vi "GDSAPI_CreateClass.vi"(7 "KeepLvClassRefOpen(False)":bool, 8 "error in (no error)":errorcluster, 9 "ClassIcon(Random colors are used if not wired)":T1, 10 "CreateClassType":T3={"ClassProvider"=enum."GOOP-3(By reference)", "NewClassFolder"=path "", "ParentLvClassFilePath"=path "", "ClassName"="", "ClassDescription"="", "ClassTemplate"=enum."Standard"}, 11 "ProjectItemToCraeteClassUnder":refnum<vi>) -> (0 "error out":errorcluster, 2 "LVClassLibraryRefnum":refnum<vi>, 3 "LvClassFileOut":path)   [LabVIEW 2016]
doc: "NOT Yet implemented"
uses:
  <resource>/Framework/Providers/Open_GDS/API/GDSAPI_CreateClassType.ctl
  <resource>/Framework/Providers/Open_GDS/API/GDSAPI_SubVIs/GDSAPI_ClassProviderType.ctl
  <resource>/Framework/Providers/Open_GDS/API/GDSAPI_SubVIs/GDSAPI_ClassTemplateType.ctl
  <resource>/Framework/Providers/Open_GDS/API/GDSAPI_SubVIs/GDSAPI_ClassIcon.ctl
  <resource>/Framework/Providers/Open_GDS/API/GDSAPI_SubVIs/GDSAPI_ClassIconType.ctl
  <resource>/Framework/Providers/Open_GDS/ClassProviders/Provider_BaseClassInterface/CreateClassData.ctl
  <resource>/Framework/Providers/Open_GDS/ClassProviders/Common/LvIcon_class/GDSLvIcon_ClassColorTypes.ctl
  <resource>/Framework/Providers/Open_GDS/ClassProviders/Common/ScriptingFunctions/Scripting_ConnectorPanePatternType.ctl
  <resource>/Framework/Providers/Open_GDS/ClassProviders/Provider_LvNativeClass/ClassWriterNative_class/ClassWriterNative.lvclass
  <resource>/Framework/Providers/Open_GDS/ClassProviders/Provider_EndevoGOOP300/ClassWriterGOOP300_class/ClassWriterGOOP300.lvclass
  C:/Program Files (x86)/National Instruments/LabVIEW 2016/resource/Framework/Providers/Open_GDS/ClassProviders/Provider_LvNativeClass/ClassWriterNative_class/ClassWriterNative.lvclass
  <resource>/Framework/Providers/Open_GDS/ClassProviders/Provider_EndevoGOOP400/ClassWriterGOOP400_class/ClassWriterGOOP400.lvclass
  <resource>/Framework/Providers/Open_GDS/ClassProviders/Provider_BaseClassInterface/ClassWriter_class/ClassWriter.lvclass
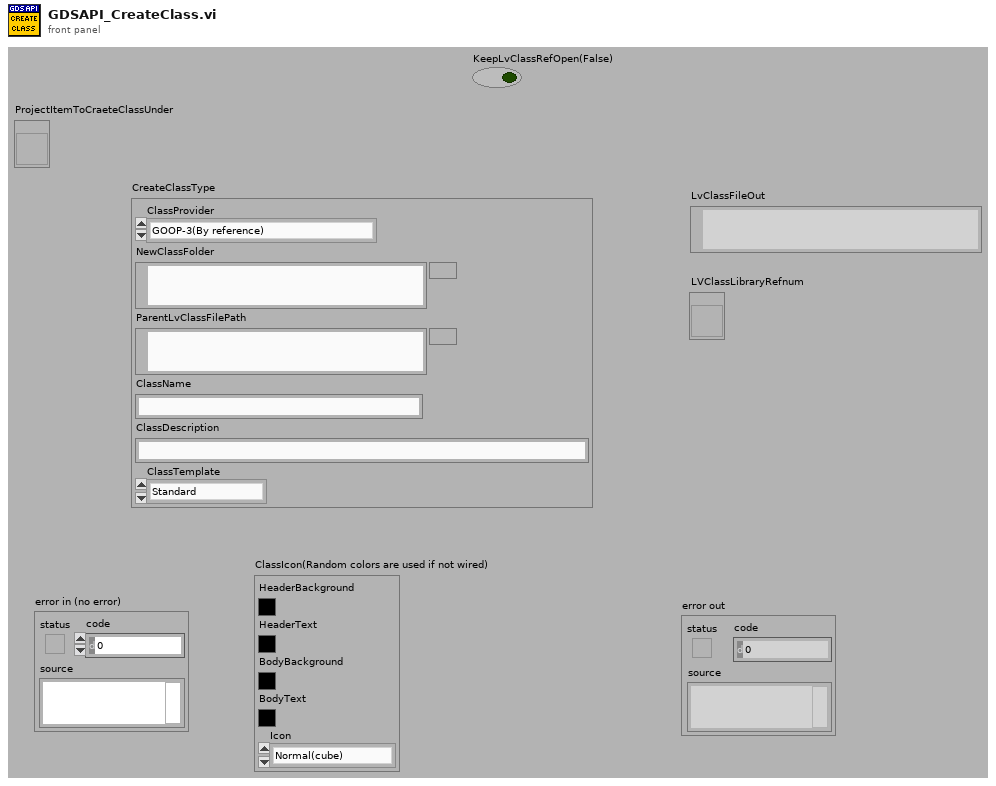
[diagram p1: front panel]
types:
  T1 = typedef "GDSAPI_ClassIcon.ctl" = cluster{"HeaderBackground":u32, "HeaderText":u32, "BodyBackground":u32, "BodyText":u32, "Icon":T2}
  T2 = typedef "GDSAPI_ClassIconType.ctl" = enum16{"Normal(cube)", "Actor", "Message", "Interface"}
  T3 = typedef "GDSAPI_CreateClassType.ctl" = cluster{"ClassProvider":T4, "NewClassFolder":path, "ParentLvClassFilePath":path, "ClassName":string, "ClassDescription":string, "ClassTemplate":T5}
  T4 = typedef "GDSAPI_ClassProviderType.ctl" = enum16{"LabVIEW Native(By value)", "GOOP-3(By reference)", "GOOP-4(By reference)"}
  T5 = typedef "GDSAPI_ClassTemplateType.ctl" = enum16{"Standard", "Singleton", "Interface(By Aggregation)", "Interface(By VI Server)"}
  T6 = typedef "GDSLvIcon_ClassColorTypes.ctl" = cluster{"Frame":u32, "Header Text Color":u32, "Header Background":u32, "BodyBackgroundPublic":u32, "BodyBackgroundProtected":u32, "BodyBackgroundPrivate":u32, "Body Text Color":u32, "Frame thickness":u8, "ProtectedPrivateSame":bool, "Icon Header Size":u8, "Font Compression":enum16{"Auto", "On", "Off"}, "CapitalOnly":bool}
  T7 = cluster{"Colors":T6, "LibraryIcon":cluster{"LibraryIcon":string, "HeaderRows(1)":u8}}
  T8 = typedef "ClassWriter.lvclass/CreateClassData.ctl" = cluster{"ClassName":string, "ClassFolder":path, "ClassDescription":string, "ClassTemplateOptions":string, "BaseClass(ProjectStringPath or LvClassFilePath)":variant, "ExtraCreateParameters":variant, "FolderSuffix":string}
  T9 = typedef "Scripting_ConnectorPanePatternType.ctl" = u16
  T10 = typedef "GDSLvCLass_ClassSettingsType.ctl" = cluster{"ClassProviderName":string, "ClassTemplateUsed":string, "ClassTemplateVersion":string, "ClassDescription":string, "PlugIns":T11[], "ConnectorPanePattern":string}
  T11 = typedef "GDSLvClass_PlugIn.ctl" = cluster{"Type":T12, "ID":string, "Version":string, "Path":path, "Name":string, "Data":variant}
  T12 = typedef "GDSLvClass_PlugInTypes.ctl" = enum16{"DesignPattern", "MethodTypes"}
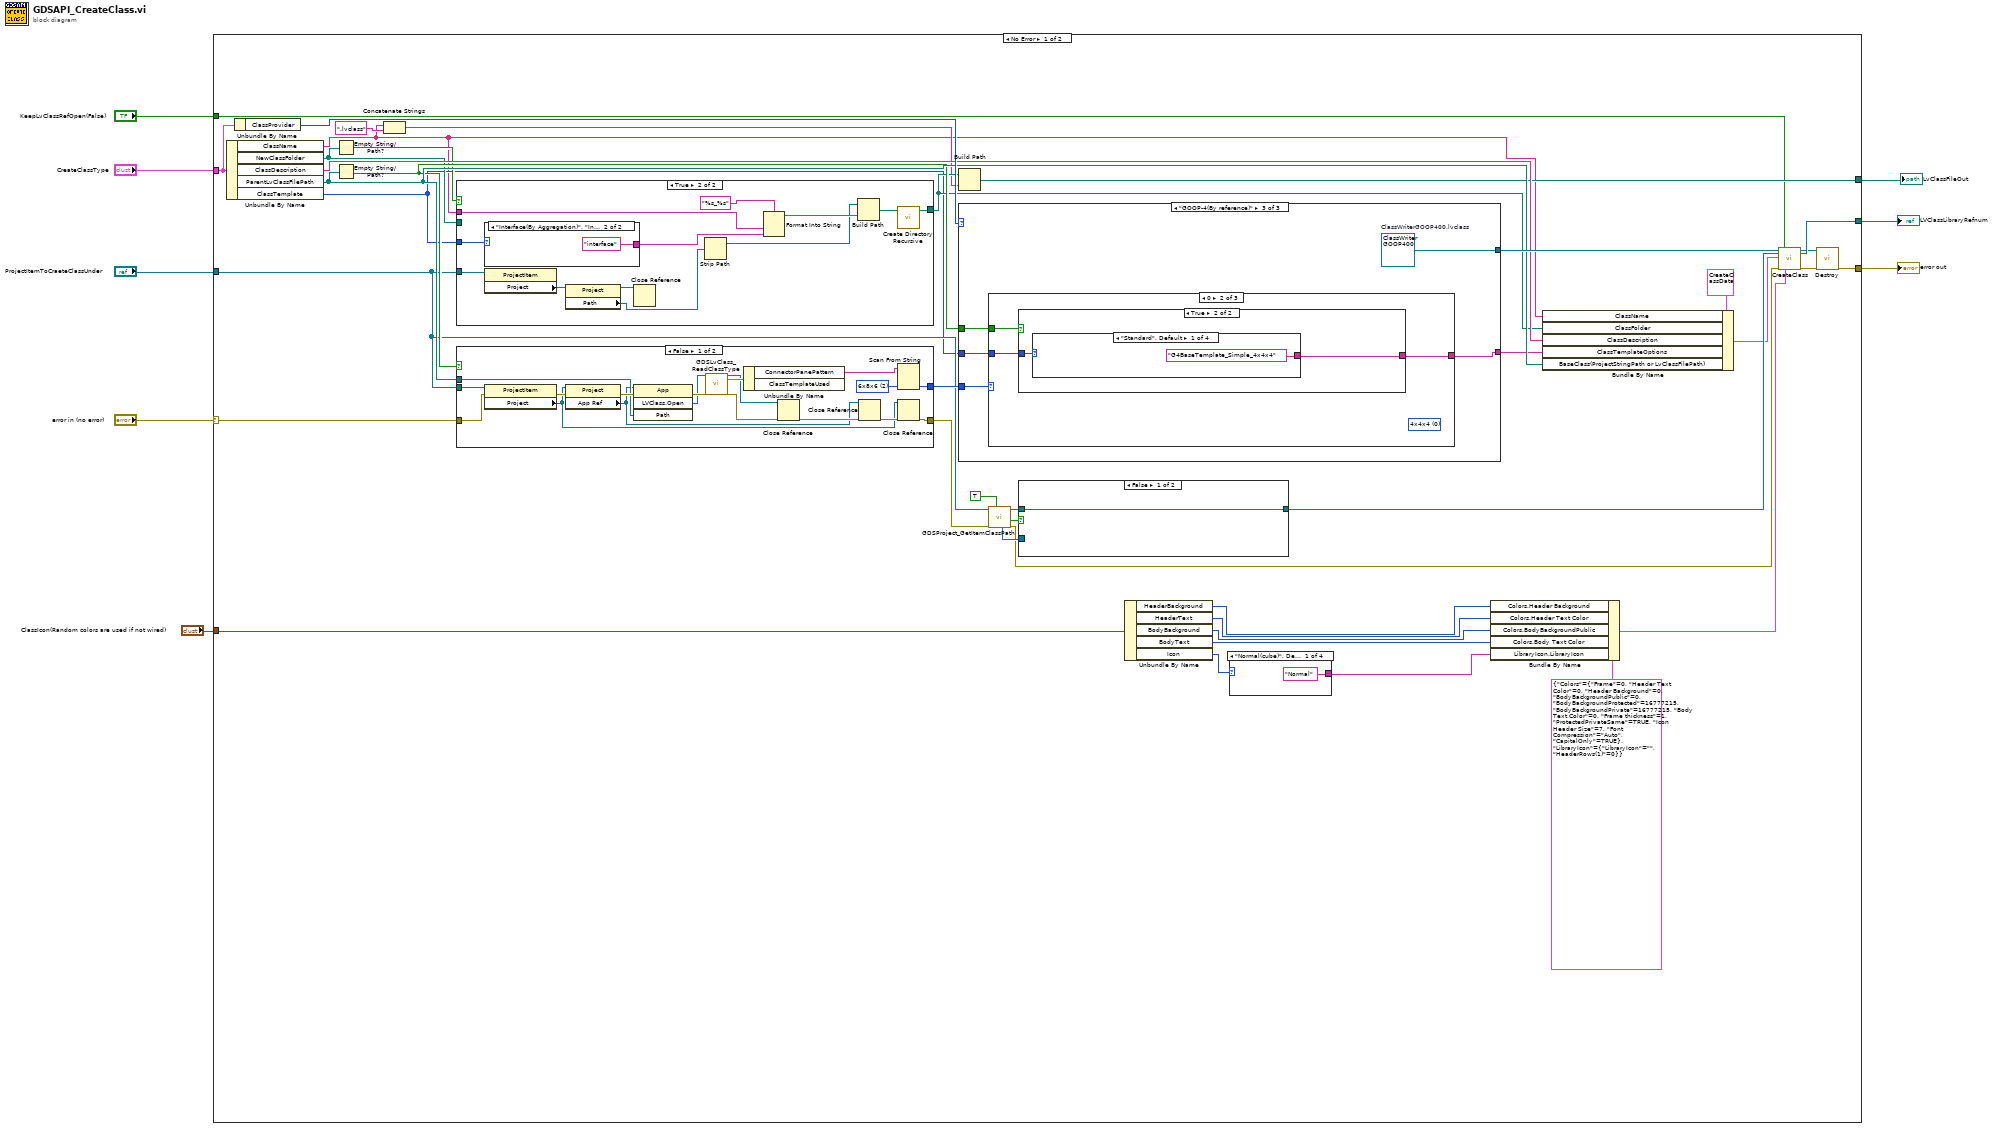
[diagram p0: block diagram]
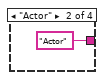
[diagram p2: hidden frame]
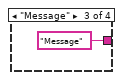
[diagram p3: hidden frame]
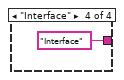
[diagram p4: hidden frame]
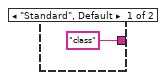
[diagram p6: hidden frame]
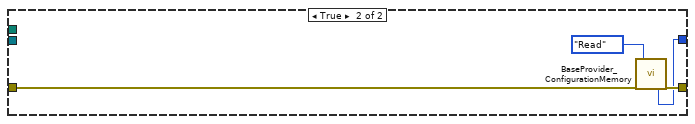
[diagram p7: hidden frame]
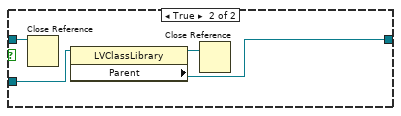
[diagram p8: hidden frame]
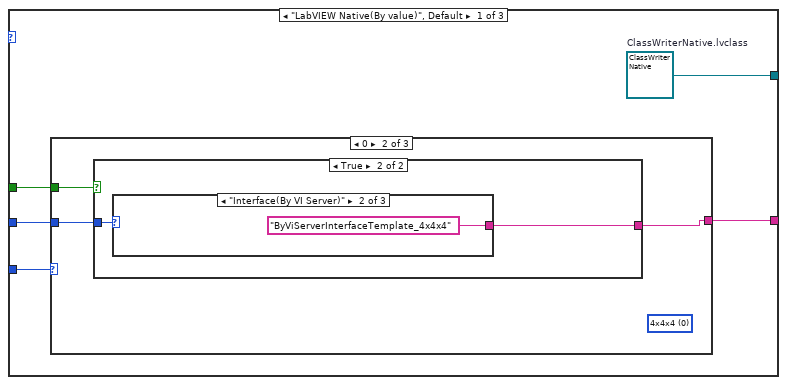
[diagram p9: hidden frame]
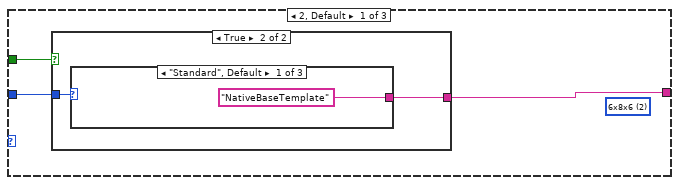
[diagram p10: hidden frame]
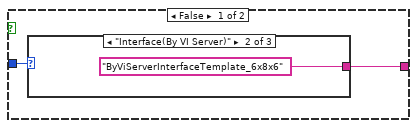
[diagram p11: hidden frame]
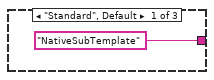
[diagram p12: hidden frame]
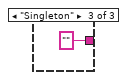
[diagram p13: hidden frame]
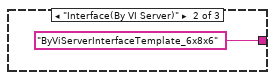
[diagram p14: hidden frame]
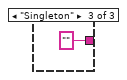
[diagram p15: hidden frame]
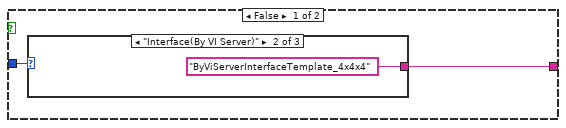
[diagram p16: hidden frame]
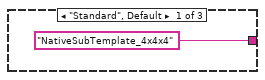
[diagram p17: hidden frame]
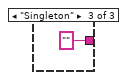
[diagram p18: hidden frame]
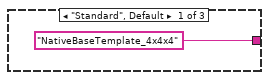
[diagram p19: hidden frame]
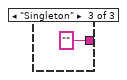
[diagram p20: hidden frame]
diagram:
  n1 = case shown="No Error" "error in (no error)" {
    selector: "error in (no error)" -> [w9 w234]
    tunnel: [w43 _] -> w8
    tunnel: [w39 w234] -> w7
    tunnel: "CreateClassType" -> [w37 _]
    tunnel: "ProjectItemToCraeteClassUnder" -> [w28 _]
    tunnel: "ClassIcon(Random colors are used if not wired)" -> [w25 _]
    tunnel: [w15 _] -> w3
    tunnel: "KeepLvClassRefOpen(False)" -> [w10 _]
    frame No Error {
      n2 = Unbundle By Name(w37) -> ("ClassName"=w13:string, "NewClassFolder"=w29:path, "ClassDescription"=w36:string, "ParentLvClassFilePath"=w34:path, "ClassTemplate"=w14:T5)
      n3 = Unbundle By Name(w37) -> ("ClassProvider"=w41:T4)
      n4 = Empty String/Path?(string/path=w29) -> (empty?=w30:bool)
      n5 = Empty String/Path?(string/path=w34) -> (empty?=w32:bool)
      n6 = Concatenate Strings(w13, ".lvclass" ("string")) -> (w16:string)
      n7 = case shown="True" w30 {
        tunnel: w29 -> [w54 _]
        tunnel: [w54 w58] -> w18
        tunnel: w28 -> [_ w66]
        tunnel: w14 -> [_ w57]
        tunnel: w13 -> [_ w55]
        frame False {
        }
        frame True {
          n8 = case shown="\"Interface(By Aggregation)\", \"Interface(By VI Server)\"" w57 {
            tunnel: ["class" ("format string") "interface" ("format string")] -> w56
            frame "Standard", Default {
            }
            frame "Interface(By Aggregation)", "Interface(By VI Server)" {
            }
          }
          n9 = property class="ProjectItem"(reference=w66) -> ("Project"=w65:refnum<vi>)  [unwired: 1 in, 2 out]
          n10 = property class="Project"(reference=w65) -> (reference out=w63:refnum<vi>, "Path"=w64:path)  [unwired: 1 in, 1 out]
          n11 = Close Reference(reference=w63) -> ()  [unwired: 1 in, 1 out]
          n12 = Strip Path(path=w64) -> (stripped path=w59:path)  [unwired: 1 out]
          n13 = Format Into String(format string="%s_%s", w55, w56) -> (resulting string=w61:string)  [unwired: 2 in, 1 out]
          n14 = Build Path(base path=w59, name or relative path=w61) -> (appended path=w60:path)
          n15 = call <vilib>:"Create Directory Recursive.vi"("directory"=w60) -> ("directory copy"=w58:path)  [unwired: 4 in, 2 out]
        }
      }
      n16 = case shown="False" w32 {
        tunnel: [w69 w89] -> w35
        tunnel: [w83 w88] -> w33
        tunnel: w28 -> [w82 _]
        tunnel: w9 -> [w81 w87]
        tunnel: w34 -> [w76 _]
        frame False {
          w84 = T9 2 items=["4x4x4", "5x6x5", "6x8x6"] ("Pattern")
          n17 = property class="ProjectItem"(reference=w82, error in=w81) -> (error out=w80:errorcluster, "Project"=w71:refnum<vi>)  [unwired: 1 out]
          n18 = property class="Project"(reference=w71, error in=w80) -> (error out=w79:errorcluster, "App Ref"=w73:refnum<vi>)  [unwired: 1 out]
          n19 = invoke class="App" method="LVClass.Open"(reference=w73, error in=w79, "Path"=w76) -> (error out=w78:errorcluster, "LVClass.Open"=w77:refnum<vi>)  [unwired: 1 in, 2 out]
          n20 = call <resource>:"GDSLvClass_ReadClassType.vi"("Class Refnum In"=w77, "error in (no error)"=w78) -> ("Class Refnum Out"=w75:refnum<vi>, "ClassSettings"=w86:T10, "error out"=w70:errorcluster)  [unwired: 15 in]
          n21 = Unbundle By Name(w86) -> ("ConnectorPanePattern"=w85:string)  [unwired: 1 out]
          n22 = Close Reference(reference=w75, error in (no error)=w70) -> (error out=w74:errorcluster)
          n23 = Close Reference(reference=w73, error in (no error)=w74) -> (error out=w72:errorcluster)
          n24 = Scan From String(input string=w85, default 1=w84) -> (output 1=w83:T9)  [unwired: 3 in, 3 out]
          n25 = Close Reference(reference=w71, error in (no error)=w72) -> (error out=w69:errorcluster)
        }
        frame True {
          n26 = call <resource>:"BaseProvider_ConfigurationMemory.vi"("error in (no error)"=w87, "Action"=enum16{"Read", "Load", "Save"}."Read") -> ("PatternOut"=w88:T9, "error out"=w89:errorcluster)  [unwired: 11 in, 5 out]
        }
      }
      n27 = Build Path(base path=w18, name or relative path=w16) -> (appended path=w15:path)
      n28 = case shown="\"GOOP-4(By reference)\"" w41 {
        tunnel: [w100 w144 w188] -> w42
        tunnel: w33 -> [w96 w140 w187]
        tunnel: w32 -> [w98 w142 w186]
        tunnel: w14 -> [w97 w141 w185]
        tunnel: [w99 w143 w184] -> w31
        frame "LabVIEW Native(By value)", Default {
          w100 = refnum<class "ClassWriterNative.lvclass"> refnum  # ClassWriterNative.lvclass
          n29 = case shown="0" w96 {
            tunnel: w98 -> [w103 w116 w129]
            tunnel: w97 -> [w102 w115 w128]
            tunnel: [w101 w114 w127] -> w99
            frame 2, Default {
              (unwired) T9 2 items=["4x4x4", "5x6x5", "6x8x6"] ("Pattern")
              n30 = case shown="True" w103 {
                tunnel: w102 -> [w105 w110]
                tunnel: [w104 w109] -> w101
                frame False {
                  n31 = case shown="\"Interface(By VI Server)\"" w105 {
                    tunnel: ["NativeSubTemplate" ("TemplateIdName") "ByViServerInterfaceTemplate_6x8x6" ("TemplateIdName") "" ("TemplateIdName")] -> w104
                    frame "Standard", Default {
                    }
                    frame "Interface(By VI Server)" {
                    }
                    frame "Singleton" {
                    }
                  }
                }
                frame True {
                  n32 = case shown="\"Standard\", Default" w110 {
                    tunnel: ["NativeBaseTemplate" ("TemplateIdName") "ByViServerInterfaceTemplate_6x8x6" ("TemplateIdName") "" ("TemplateIdName")] -> w109
                    frame "Standard", Default {
                    }
                    frame "Interface(By VI Server)" {
                    }
                    frame "Singleton" {
                    }
                  }
                }
              }
            }
            frame 0 {
              (unwired) T9 0 items=["4x4x4", "5x6x5", "6x8x6"] ("Pattern")
              n33 = case shown="True" w116 {
                tunnel: w115 -> [w118 w123]
                tunnel: [w117 w122] -> w114
                frame False {
                  n34 = case shown="\"Interface(By VI Server)\"" w118 {
                    tunnel: ["NativeSubTemplate_4x4x4" ("TemplateIdName") "ByViServerInterfaceTemplate_4x4x4" ("TemplateIdName") "" ("TemplateIdName")] -> w117
                    frame "Standard", Default {
                    }
                    frame "Interface(By VI Server)" {
                    }
                    frame "Singleton" {
                    }
                  }
                }
                frame True {
                  n35 = case shown="\"Interface(By VI Server)\"" w123 {
                    tunnel: ["NativeBaseTemplate_4x4x4" ("TemplateIdName") "ByViServerInterfaceTemplate_4x4x4" ("TemplateIdName") "" ("TemplateIdName")] -> w122
                    frame "Standard", Default {
                    }
                    frame "Interface(By VI Server)" {
                    }
                    frame "Singleton" {
                    }
                  }
                }
              }
            }
            frame 1 {
              (unwired) T9 1 items=["4x4x4", "5x6x5", "6x8x6"] ("Pattern")
              n36 = case shown="True" w129 {
                tunnel: w128 -> [w131 w136]
                tunnel: [w130 w135] -> w127
                frame False {
                  n37 = case shown="\"Interface(By VI Server)\"" w131 {
                    tunnel: ["NativeSubTemplate" ("TemplateIdName") "ByViServerInterfaceTemplate_6x8x6" ("TemplateIdName") "" ("TemplateIdName")] -> w130
                    frame "Standard", Default {
                    }
                    frame "Interface(By VI Server)" {
                    }
                    frame "Singleton" {
                    }
                  }
                }
                frame True {
                  n38 = case shown="\"Interface(By VI Server)\"" w136 {
                    tunnel: ["NativeBaseTemplate" ("TemplateIdName") "ByViServerInterfaceTemplate_6x8x6" ("TemplateIdName") "" ("TemplateIdName")] -> w135
                    frame "Standard", Default {
                    }
                    frame "Interface(By VI Server)" {
                    }
                    frame "Singleton" {
                    }
                  }
                }
              }
            }
          }
        }
        frame "GOOP-3(By reference)" {
          w144 = refnum<class "ClassWriterGOOP300.lvclass"> refnum  # ClassWriterGOOP300.lvclass
          n39 = case shown="0" w140 {
            tunnel: w142 -> [w147 w160 w173]
            tunnel: w141 -> [w146 w159 w172]
            tunnel: [w145 w158 w171] -> w143
            frame 2, Default {
              (unwired) T9 2 items=["4x4x4", "5x6x5", "6x8x6"] ("Pattern")
              n40 = case shown="False" w147 {
                tunnel: w146 -> [w149 w154]
                tunnel: [w148 w153] -> w145
                frame False {
                  n41 = case shown="\"Interface(By VI Server)\"" w149 {
                    tunnel: ["SubTemplate" ("TemplateIdName") "ByViServerInterfaceTemplate_6x8x6" ("TemplateIdName") "" ("TemplateIdName")] -> w148
                    frame "Standard", Default {
                    }
                    frame "Interface(By VI Server)" {
                    }
                    frame "Singleton" {
                    }
                  }
                }
                frame True {
                  n42 = case shown="\"Interface(By VI Server)\"" w154 {
                    tunnel: ["BaseTemplate" ("TemplateIdName") "SingletonTemplate" ("TemplateIdName") "ByViServerInterfaceTemplate_6x8x6" ("TemplateIdName")] -> w153
                    frame "Standard", Default {
                    }
                    frame "Singleton" {
                    }
                    frame "Interface(By VI Server)" {
                    }
                  }
                }
              }
            }
            frame 0 {
              (unwired) T9 0 items=["4x4x4", "5x6x5", "6x8x6"] ("Pattern")
              n43 = case shown="True" w160 {
                tunnel: w159 -> [w162 w167]
                tunnel: [w161 w166] -> w158
                frame False {
                  n44 = case shown="\"Interface(By VI Server)\"" w162 {
                    tunnel: ["SubTemplate_4x4x4" ("TemplateIdName") "ByViServerInterfaceTemplate_4x4x4" ("TemplateIdName") "G4SubTemplate_Singleton_4x4x4" ("TemplateIdName")] -> w161
                    frame "Standard", Default {
                    }
                    frame "Interface(By VI Server)" {
                    }
                    frame "Singleton" {
                    }
                  }
                }
                frame True {
                  n45 = case shown="\"Interface(By VI Server)\"" w167 {
                    tunnel: ["BaseTemplate_4x4x4" ("TemplateIdName") "ByViServerInterfaceTemplate_4x4x4" ("TemplateIdName") "SingletonTemplate" ("TemplateIdName")] -> w166
                    frame "Standard", Default {
                    }
                    frame "Interface(By VI Server)" {
                    }
                    frame "Singleton" {
                    }
                  }
                }
              }
            }
            frame 1 {
              (unwired) T9 1 items=["4x4x4", "5x6x5", "6x8x6"] ("Pattern")
              n46 = case shown="False" w173 {
                tunnel: w172 -> [w175 w180]
                tunnel: [w174 w179] -> w171
                frame False {
                  n47 = case shown="\"Interface(By VI Server)\"" w175 {
                    tunnel: ["SubTemplate" ("TemplateIdName") "ByViServerInterfaceTemplate_6x8x6" ("TemplateIdName") "" ("TemplateIdName")] -> w174
                    frame "Standard", Default {
                    }
                    frame "Interface(By VI Server)" {
                    }
                    frame "Singleton" {
                    }
                  }
                }
                frame True {
                  n48 = case shown="\"Interface(By VI Server)\"" w180 {
                    tunnel: ["BaseTemplate" ("TemplateIdName") "ByViServerInterfaceTemplate_6x8x6" ("TemplateIdName") "SingletonTemplate" ("TemplateIdName")] -> w179
                    frame "Standard", Default {
                    }
                    frame "Interface(By VI Server)" {
                    }
                    frame "Singleton" {
                    }
                  }
                }
              }
            }
          }
        }
        frame "GOOP-4(By reference)" {
          w188 = refnum<class "ClassWriterGOOP400.lvclass"> refnum  # ClassWriterGOOP400.lvclass
          n49 = case shown="0" w187 {
            tunnel: w186 -> [w191 w206 w221]
            tunnel: w185 -> [w190 w205 w220]
            tunnel: [w189 w204 w219] -> w184
            frame 2, Default {
              (unwired) T9 2 items=["4x4x4", "5x6x5", "6x8x6"] ("Pattern")
              n50 = case shown="False" w191 {
                tunnel: w190 -> [w193 w199]
                tunnel: [w192 w198] -> w189
                frame False {
                  n51 = case shown="\"Interface(By Aggregation)\"" w193 {
                    tunnel: ["G4SubTemplate_Simple_6x8x6" ("TemplateIdName") "ByViServerInterfaceTemplate_4x4x4" ("TemplateIdName") "G4InterfaceTemplate_6x8x6" ("TemplateIdName") "G4SubTemplate_Singleton_6x8x6" ("TemplateIdName")] -> w192
                    frame "Standard", Default {
                    }
                    frame "Interface(By VI Server)" {
                    }
                    frame "Interface(By Aggregation)" {
                    }
                    frame "Singleton" {
                    }
                  }
                }
                frame True {
                  n52 = case shown="\"Interface(By Aggregation)\"" w199 {
                    tunnel: ["G4BaseTemplate_Simple_6x8x6" ("TemplateIdName") "ByViServerInterfaceTemplate_4x4x4" ("TemplateIdName") "G4InterfaceTemplate_6x8x6" ("TemplateIdName") "G4BaseTemplate_Singleton_6x8x6" ("TemplateIdName")] -> w198
                    frame "Standard", Default {
                    }
                    frame "Interface(By VI Server)" {
                    }
                    frame "Interface(By Aggregation)" {
                    }
                    frame "Singleton" {
                    }
                  }
                }
              }
            }
            frame 0 {
              (unwired) T9 0 items=["4x4x4", "5x6x5", "6x8x6"] ("Pattern")
              n53 = case shown="True" w206 {
                tunnel: w205 -> [w208 w214]
                tunnel: [w207 w213] -> w204
                frame False {
                  n54 = case shown="\"Standard\", Default" w208 {
                    tunnel: ["G4SubTemplate_Simple_4x4x4" ("TemplateIdName") "ByViServerInterfaceTemplate_4x4x4" ("TemplateIdName") "G4InterfaceTemplate_4x4x4" ("TemplateIdName") "G4SubTemplate_Singleton_4x4x4" ("TemplateIdName")] -> w207
                    frame "Standard", Default {
                    }
                    frame "Interface(By VI Server)" {
                    }
                    frame "Interface(By Aggregation)" {
                    }
                    frame "Singleton" {
                    }
                  }
                }
                frame True {
                  n55 = case shown="\"Standard\", Default" w214 {
                    tunnel: ["G4BaseTemplate_Simple_4x4x4" ("TemplateIdName") "ByViServerInterfaceTemplate_4x4x4" ("TemplateIdName") "G4InterfaceTemplate_4x4x4" ("TemplateIdName") "G4BaseTemplate_Singleton_4x4x4" ("TemplateIdName")] -> w213
                    frame "Standard", Default {
                    }
                    frame "Interface(By VI Server)" {
                    }
                    frame "Interface(By Aggregation)" {
                    }
                    frame "Singleton" {
                    }
                  }
                }
              }
            }
            frame 1 {
              (unwired) T9 1 items=["4x4x4", "5x6x5", "6x8x6"] ("Pattern")
              n56 = case shown="True" w221 {
                tunnel: w220 -> [w223 w229]
                tunnel: [w222 w228] -> w219
                frame False {
                  n57 = case shown="\"Interface(By Aggregation)\"" w223 {
                    tunnel: ["G4SubTemplate_Simple_5x6x5" ("TemplateIdName") "ByViServerInterfaceTemplate_4x4x4" ("TemplateIdName") "G4InterfaceTemplate_6x8x6" ("TemplateIdName") "G4SubTemplate_Singleton_5x6x5" ("TemplateIdName")] -> w222
                    frame "Standard", Default {
                    }
                    frame "Interface(By VI Server)" {
                    }
                    frame "Interface(By Aggregation)" {
                    }
                    frame "Singleton" {
                    }
                  }
                }
                frame True {
                  n58 = case shown="\"Interface(By Aggregation)\"" w229 {
                    tunnel: ["G4BaseTemplate_Simple_5x6x5" ("TemplateIdName") "ByViServerInterfaceTemplate_4x4x4" ("TemplateIdName") "G4InterfaceTemplate_6x8x6" ("TemplateIdName") "G4BaseTemplate_Singleton_5x6x5" ("TemplateIdName")] -> w228
                    frame "Standard", Default {
                    }
                    frame "Interface(By VI Server)" {
                    }
                    frame "Interface(By Aggregation)" {
                    }
                    frame "Singleton" {
                    }
                  }
                }
              }
            }
          }
        }
      }
      n59 = call <resource>:"GDSProject_GetItemClassPath.vi"("ReturnRefToClass(False)"=TRUE, "error in"=w35, "ProjectItemRefIn"=w28) -> ("error out"=w40:errorcluster, "LvCLassFound"=w48:bool, "ProjectItemRefOut"=w47:refnum<vi>, "LvClassRef"=w45:refnum<vi>)  [unwired: 3 in, 2 out]
      n60 = case shown="False" w48 {
        tunnel: w47 -> [w91 w95]
        tunnel: [w91 w93] -> w46
        tunnel: w45 -> [_ w94]
        frame False {
        }
        frame True {
          n61 = Close Reference(reference=w95) -> ()  [unwired: 1 in, 1 out]
          n62 = property class="LVClassLibrary"(reference=w94) -> (reference out=w92:refnum<vi>, "Parent"=w93:refnum<vi>)  [unwired: 1 in, 1 out]
          n63 = Close Reference(reference=w92) -> ()  [unwired: 1 in, 1 out]
        }
      }
      n64 = Unbundle By Name(w25) -> ("HeaderBackground"=w24:u32, "HeaderText"=w23:u32, "BodyBackground"=w22:u32, "BodyText"=w21:u32, "Icon"=w20:T2)
      n65 = case shown="\"Normal(cube)\", Default" w20 {
        tunnel: ["Normal" ("LibraryIcon.LibraryIcon") "Actor" "Message" "Interface"] -> w19
        frame "Normal(cube)", Default {
        }
        frame "Actor" {
        }
        frame "Message" {
        }
        frame "Interface" {
        }
      }
      n66 = Bundle By Name(cluster=T7 {"Colors"={"Frame"=0, "Header Text Color"=0, "Header Background"=0, "BodyBackgroundPublic"=0, "BodyBackgroundProtected"=16777215, "BodyBackgroundPrivate"=16777215, "Body Text Color"=0, "Frame thickness"=1, "ProtectedPrivateSame"=TRUE, "Icon Header Size"=7, "Font Compression"=enum."Auto", "CapitalOnly"=TRUE}, "LibraryIcon"={"LibraryIcon"="", "HeaderRows(1)"=0}} ("output cluster"), "Colors.Header Background"=w24, "Colors.Header Text Color"=w23, "Colors.BodyBackgroundPublic"=w22, "Colors.Body Text Color"=w21, "LibraryIcon.LibraryIcon"=w19) -> (w26:T7)
      n67 = Bundle By Name(cluster=T8 {"ClassName"="", "ClassFolder"=path "", "ClassDescription"="", "ClassTemplateOptions"="", "BaseClass(ProjectStringPath or LvClassFilePath)"=variant, "ExtraCreateParameters"=variant, "FolderSuffix"=""} ("CreateClassData"), "ClassName"=w13, "ClassFolder"=w18, "ClassDescription"=w36, "ClassTemplateOptions"=w31, "BaseClass(ProjectStringPath or LvClassFilePath)"=w34) -> (w38:T8)
      n68 = call-dynamic "CreateClass.vi"("ClassWriterNative"=w42, "ProjectTreePosition(String or Project Item Ref)"=w46, "CreateClassData"=w38, "error in (no error)"=w40, "KeepLvClassRefOpen(False)"=w10, "HeaderToApply (take from VIRef or /use 2D-8bit header, Ignored if not wired)"=w26) -> ("ClassWriterNative"=w12:refnum<class "ClassWriterNative.lvclass">, "LVClassLibraryRefnum"=w43:refnum<vi>, "error out"=w44:errorcluster)  [unwired: 10 in, 1 out]
      n69 = call-dynamic "Destroy.vi"("ClassWriterNative"=w12, "error in (no error)"=w44) -> ("error out"=w39:errorcluster)  [unwired: 17 in]
    }
    frame Error {
    }
  }
  "error out" <- w7
  "LvClassFileOut" <- w3
  "LVClassLibraryRefnum" <- w8
